vi "Translator.Translate.StepStatus (NoError).vi"(9 "Arguments":variant[](array[variant]), 10 "msg":T1) -> (2 "Translated Msg":string)   [LabVIEW 2013]
uses:
  Translator.Message.ctl
  Translator.Global.vi
panel:
  out "error out":errorcluster
  in  "error in (no error)":errorcluster
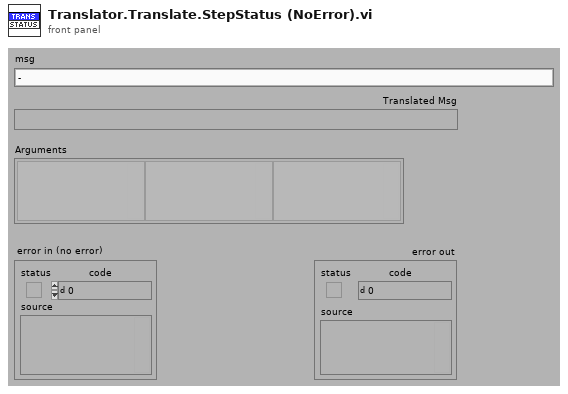
[diagram p1: front panel]
types:
  T1 = typedef "Translator.Message.ctl" = enum16{"-", "Log out", "Log in", "Shutdown", "Cancel", "Start", "Error %d >> %s >> %s", "Starting %s", "Quitting %s", "User %s level %s added", "User %s level %s deleted", "User %s level %s changed to %s", "Initializing...", "Quitting...", "Loading...", "Shutdown production line?", "Calibration", "Log out?", "System", "All", "IDLE", "Translating...%s", "Positioning press...", "Positioning unit...", "Needle left...", "Needle up...", "Needle right...", "Needle down...", "Needle left & down...", "Wrong orientation", "Not found", "Put pin in screw hole pos 2", "Put pin in home position", "Set screwdrivers in home position", "Set vertical screwdriver in home pos", "Set horizontal screwdriver in home pos", "Set vertical screwdriver in pos 1", "Set vertical screwdriver in pos 2", "Set horizontal screwdriver in pos 1", "Set horizontal screwdriver in pos 2", "Start tightening", "Move to start position", "Slide drawer", "Slide out drawer", "Slide drawer and close door", "Press start button", "Pressing...", "Pressing %d...", "Releasing...", "Releasing %d...", "Insert guiding column", "Insert guiding column and ring", "Insert spring", "Insert piston and ring, then slide the drawer and close door", "Press service button...", "Insert body plug into vacuum generator", "Wait for stabilize sensor signal", "Wrong position", "Wrong piston position or piston missing", "Ring missing", "Leak too large", "Alarm %s", "Guiding ring bottom", "Internal seal bottom", "Guiding ring top", "Internal seal top", "Ending", "Restart is required to translate the application! Do you want to restart the PC?", "Restart cancelled. Be aware that some controls may not be fully translated until you restart the application.", "New version available!", "The software is up-to-date", "PC software will be updated after rebooting the PC. Do you want to reboot now?", "RT software will be updated. Make sure that no process is running. Do you want to reboot RT now?", "Updating RT firmware. Please wait...", "Update failed: %s", "Rebooting...", "Rebooting RT. Please wait...", "RT updated to version %s", "Timeout error during update. Check if RT is working", "Closing stations...", "Service Option not available in this station!", "Piston", "Body", "Bearing", "Bracket", "Spring", "Lace", "Sensor", "Plug", "Station 1", "Station 2", "Station 3", "Station 4", "Station 5", "Station 6", "Accept & Run", "Run old configuration", "Run", "Skip", "Abort", "Confirm Alarm", "Hardware not ready", "Station powering on...", "Slide drawer to begin station initialization", "Release service mode to begin station initialization", "Close door to begin station initialization", "Press Start to begin station initialization", "Take out the product to begin station initialization", "Station initializing...", "Table position referencing...", "Press Run button to start new order", "Scan new order", "Call maintanance to solve problems!", "Insert %s", "Insert product", "Close door", "Press start", "Station could not be initialized: Emergency circuit", "Please wait...", "Checking configuration...", "Checking product...", "Sequence beginning...", "Sequence running...", "Sequence ending...", "Station shutting down...", "Take out the product", "Open door", "Confirm error with red button", "Sequence critical error. Enter service mode...", "Position reached", "Force reached", "Code already printed", "Body not present", "Piston not present", "DB: Incorrect settings", "DB: Initializing...", "DB: ERR%d >> %s", "DB: OK", "DB: Piston not completed in previous station", "DB: Body not completed  in previous station", "DB: Piston already processed in next station", "DB: Body already processed in next station", "Daq: DI #%d and #%d have share the same resource", "Daq: DO #%d and #%d have share the same resource", "Daq: DIO Incorrect settings", "Daq: AI Incorrect settings", "Daq: DIO Initializing...", "Daq: AI Initializing...", "Daq: DIO ERR%d >> %s", "Daq: AI ERR%d >> %s", "Daq: DIO OK", "Daq: AI OK", "Daq: Air pressure off", "Daq: Air pressure on", "Daq: Unable to switch on air pressure", "Daq: Unable to switch off air pressure", "Daq: CenterMarker not supported in the station", "Daq: LeakTestExhaust not supported in the station", "Daq: Unable to move LeakTestExhaust to %s position. Air pressure off", "Daq: GuidingColumn not supported in the station", "Daq: Unable to move GuidingColumn to %s position. Timeout", "Daq: Unable to move GuidingColumn to %s position. Air pressure off", "Daq: SpringSensor not supported in the station", "Daq: Unable to move SpringSensor to %s position. Timeout", "Daq: Unable to move SpringSensor to %s position. Air pressure off", "Daq: Unable to move SpringSensor to %s position. Drawer not in open position", "Daq: Connector not supported in the station", "Daq: Unable to move Connector to %s position. Timeout", "Daq: Unable to move Connector to %s position. Air pressure off", "Daq: Unable to move Connector to %s position. Drawer not in close position", "Daq: BodyPlug not supported in the station", "Daq: Unable to move BodyPlug to %s position. Timeout", "Daq: Unable to move BodyPlug to %s position. Air pressure off", "Daq: VerticalScrewPos1Block not supported in the station", "Daq: Unable to move VerticalScrewPos1Block to %s position. Timeout", "Daq: Unable to move VerticalScrewPos1Block to %s position. Air pressure off", "Daq: Stamp not supported in the station", "Daq: Unable to move Stamp to %s position. Timeout", "Daq: Unable to move Stamp to %s position. Air pressure off", "Daq: Vacuum Generator not supported in the station", "Daq: Unable to set Vacuum Generator to %s position. Timeout", "Daq: Unable to set Vacuum Generator to %s position. Air pressure off", "Daq: MiddlePositionLock not supported in the station", "Daq: Unable to move MiddlePositionLock to %s position. Timeout", "Daq: Unable to move MiddlePositionLock to %s position. Air pressure off", "Daq: Unable to move MiddlePositionLock to %s position. Emergency circuit", "Daq: Unable to move MiddlePositionLock to %s position. InternalSealings not in position Right", "Daq: Unable to move MiddlePositionLock to %s position. InternalSealings in position Middle", "Daq: InternalSealings not supported in the station", "Daq: Unable to move InternalSealings to %s position. Timeout", "Daq: Unable to move InternalSealings to %s position. Air pressure off", "Daq: Unable to move InternalSealings to %s position. Emergency circuit", "Daq: Unable to move InternalSealings to %s position. Motors in wrong position", "Daq: Grease pump off", "Daq: Grease level ok", "Daq: Grease level low", "Daq: Grease level critical low", "Scanner Piston: Incorrect settings", "Scanner Piston: Initializing...", "Scanner Piston: ERR%d >> %s", "Scanner Piston: Internal error %d", "Scanner Piston: OK", "Scanner Body: Incorrect settings", "Scanner Body: Initializing...", "Scanner Body: ERR%d >> %s", "Scanner Body: Internal error %d", "Scanner Body: OK", "Cam%d: Incorrect settings", "Cam%d: Initializing...", "Cam%d: ERR%d >> %s", "Cam%d: OK", "Cam%d: Unable to start acquisition. Camera not initialized", "Tox: Incorrect settings", "Tox: Initializing...", "Tox: Disabled", "Tox: ERR%d >> %s", "Tox: Process error %d", "TOX: Referencing...", "Tox: OK", "Tox: Unable to move to %s position. Emergency circuit", "Tox: Unable to move to %s position. Unit in work position.", "Tox: Unable to move to %s position. Unit needle in work position", "Tox: Unable to move to %s position. Printing unit in work position", "Tox: Unable to move to %s position. Festo servo motor in work position", "Tox: Unable to move to %s position. Table not in work position", "Tox: Unable to move to %s position. Internal Error", "Tox: Unable to move to %s position. Timeout", "PrintUnit: Incorrect settings", "PrintUnit: Initializing...", "PrintUnit: ERR%d >> %s", "PrintUnit: %s", "PrintUnit: OK", "PrintUnit: Internal Error. STX byte error 0x%02X", "PrintUnit: Internal Error. Unknown ack answer 0x%02X", "PrintUnit: Internal Error. Max number of read retries exceeded", "PrintUnit: Internal Error. Max number of write retries exceeded", "PrintUnit: Internal Error. Clear RX timeout", "PrintUnit: Internal Error. Object ID: read \"%s\" expected \"%s\". bData = %d. %s", "PrintUnit: Internal Error. MSG CMD %s", "PrintUnit: Unable %s move to %s position. Emergency circuit", "PrintUnit: Unable %s move to %s position. Air pressure off", "PrintUnit: Unable %s move to %s position. Tox press not in home position", "PrintUnit: Unable %s move to %s position. Timeout", "PrintUnit: Not supported in the station", "PrintUnit: Printing start alarm: %s", "PrintUnit: Printer did not accept the text (%s, %s)", "PrintUnit: Printing end alarm: %s", "PrintUnit: Printing ended unexpectedly", "PrintUnit: Printing start timeout", "PrintUnit: Printing end timeout", "Unit: Unable to move to %s position. Emergency circuit", "Unit: Unable to move to %s position. Air pressure off", "Unit: Unable to move to %s position. Timeout", "Unit: Unable to move to %s position. Table not in work position", "Unit: Unable to move to %s position. Tox not in right position", "Unit: Unable to move to %s position. Motors in wrong position", "Unit: Not supported in the station", "Unit: Needle move not supported in the station", "Unit: Unable to move needle. Air pressure off", "Unit: Unable to move Needle%d to %s position. Timeout", "Unit: Unable to move Needle%d to %s position. Air pressure off", "Unit: Unable to move Needle %s to %s position. Timeout", "Unit: Unable to move Needle %s to %s position. Air pressure off", "Unit: Unable to open Needle%d to %s position. Timeout", "Unit: Unable to open Needle%d to %s position. Air pressure off", "Unit: Needle open not supported in the station", "Unit: Unable to open needle. Air pressure off", "Ateq: Incorrect settings", "Ateq: Initializing...", "Ateq: ERR%d >> %s", "Ateq: Internal alarm", "Ateq: OK", "Ateq: Aborted. Emergency Circuit", "Ateq: Aborted.Air pressure off", "Ateq: Aborted. Timeout", "Stanley Horiz: Incorrect settings", "Stanley Vert: Incorrect settings", "Stanley Horiz: Initializing...", "Stanley Vert: Initializing...", "Stanley Horiz: ERR%d >> %s", "Stanley Vert: ERR%d >> %s", "Stanley Horiz: Alarm %s", "Stanley Vert: Alarm %s", "Stanley Horiz: OK", "Stanley Vert: OK", "Festo%d: Incorrect settings", "Festo%d: Initializing...", "Festo%d: Reference missing", "Festo%d: Voltage missing", "Festo%d: ERR%d >> %s", "Festo%d: Unable to move. Emergency circuit", "Festo%d: Unable to move. Unit in work position", "Festo%d: Unable to move. Unit needle in work position", "Festo%d: Unable to move. Tox press not in repositioning or home position", "Festo%d: Unable to move. Table not in work position", "Festo%d: Unable to move. Festo2 not in work position", "Festo%d: Unable to move. Drawer not in position", "Festo%d: Unable to move. Door not closed", "Festo%d: Unable to move.", "Festo%d: Unable to home.", "Festo%d: Aborted. Emergency circuit", "Festo%d: Aborted. Timeout", "Festo%d: Dislocation not reached force nor position", "Festo%d: Work position not reached", "Festo%d: Destination position not reached %.2f", "Festo%d: Destination position or force not reached %.2f", "Festo%d: Press position not reached", "Festo%d: Final position not reached", "Festo%d: Leak position not reached", "Festo%d: OK", "Festo%d: Internal error", "Stober%d: Incorrect settings", "Stober%d: Initializing...", "Stober%d: Disabled", "Stober%d: Not referenced", "Stober%d: Referencing...", "Stober%d: ERR%d >> %s", "Stober%d: OK", "Stober%d: Internal error %s", "Stober%d: Unable to reference", "Stober%d: Unable to home", "Stober%d: Unable to move", "Stober%d: Unable to move. Motor not initialized", "Stober%d: Unable to move. Motor not referenced", "Stober%d: Unable to move. Motor busy referencing", "Stober%d: Unable to move. Emergency circuit", "Stober%d: Unable to move. Table locked", "Stober%d: Unable to move. Festo1 not in Home position", "Stober%d: Unable to move. Festo2 not in Home position", "Stober%d: Unable to move. Festo3 in Work position", "Stober%d: Unable to move. Festo4 not in Home position", "Stober%d: Unable to move. Festo5 not in Home position", "Stober%d: Aborted. Emergency circuit", "Stober%d: Aborted. Timeout", "Stober%d: Destination position not reached", "Table: Unable to set ElectricalLock to %s position. Emergency circuit", "Table: Unable to set ElectricaLock to %s position. Drawer not in position", "DrawerLockClose not supported", "DrawerLockOpen %s timeout", "Table: Unable to move Drawer to %s position. Timeout", "Table: Unable to move Drawer to %s position. Air pressure off", "Table: Drawer move not supported in the station", "Rotation table unlocked", "Rotation table locked", "Table: not supported in the station", "Table: DraweOpenLock not supported in the station", "Table: DraweCloseLock not supported in the station", "Table: Unable to set DrawerOpenLock to %s position. Timeout", "Table: Unable to set DrawerOpenLock to %s position. Emergency circuit", "Table: Unable to set DrawerOpenLock to %s position. Air pressure off", "Table: Unable to set DrawerOpenLock to %s position. Drawer not in intermediate position", "Table: Unable to set DrawerOpenLock to %s position. Drawer not in open/intermediate position", "Table: Unable to set DrawerOpenLock to %s position. Screwdrivers not in Home position", "Table: Unable to set DrawerCloseLock to %s position. Timeout", "Table: Unable to set DrawerCloseLock to %s position. Emergency circuit", "Table: Unable to set DrawerCloseLock to %s position. Air pressure off", "Table: Unable to set DrawerCloseLock to %s position. Drawer not in close position", "Table: Lock not supported in the station", "Table: Unable to lock at position %s. Emergency circuit", "Table: Unable to lock at position %s. Air pressure off", "Table: Unable to lock at position %s. Out of position", "Table: Unable to lock at position %s. Timeout", "Table: Unable to move to %s position. Timeout", "Table: Unable to move to %s position. Press not in home position", "Table: Unable to move to %s position. Emergency circuit", "Table: Unable to move to %s position. Air pressure off", "Table: Unable to move to %s position. Unit not in home position", "Table: Unable to move to %s position. Connector not in home position", "Table: Unable to move to %s position. Stamp not in home position", "Table: Unable to move to %s position. Motor not in home position", "Table: unable to move to %s position. Invalid motor %d state (%s)", "Seq: Unable to start. Invalid motor %d state (%s)", "Seq: Unable to start. Piston already has code %s", "Seq: Unable to start. Invalid piston position %.2f", "Seq: Unable to find reference position of motor %d", "Seq: Unable to rotate table. %s", "Seq: Greasing needle open activation signal timeout", "Seq: Greasing flow too high", "Seq: Greasing process failed to start because of motor", "Seq: Homing after process failed", "Seq: Emergency circuit abort", "Seq: Tightening aborted", "Seq: Analog signal stabilizing timeout", "Seq: Incorrect sequence settings", "Seq: Piston not assembled", "Seq: Incorrect Part Number", "Station: Initializing...", "Station: Incorrect settings", "Station: %s ERR%d >> %s", "Station: OK", "Station: Process running...", "Station: Unable to initialized: Emergency circuit"}
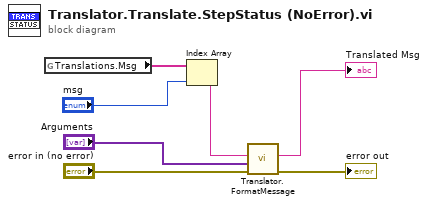
[diagram p0: block diagram]
diagram:
  n1 = global read "Translator.Global.vi" "Translations.Msg"() -> (w4:string[])
  n2 = Index Array(array=w4, index="msg") -> (element=w2:string)
  n3 = call "Translator.FormatMessage.vi"("error in (no error)"="error in (no error)", "Arguments"="Arguments", "Msg"=w2) -> ("error out"=→"error out":errorcluster, "Translated Msg"=→"Translated Msg":string)  [unwired: 7 in]
